vi "16T_Split_Cluster.vi"(0 "16 T Magnet control":T3={"Clamp"=FALSE, "Switch Heater"=FALSE, "Go to Zero"=FALSE, "Go to set"=FALSE, "Go to Hold"=FALSE, "Clamped"=FALSE, "Quenched"=FALSE, "Rate limit"=FALSE, "Persistent"=FALSE, "Hold"=FALSE, "Set"=FALSE, "Zero"=FALSE, "Magnet (T)"=0.0, "Leads (T)"=0.0, "Magnet T (K)"=3.4572, "Switch"=FALSE, "Setpoint (T)"=3.4572, "Rate (T/min)"=0.0, "Select"=FALSE, "Sweeping"=FALSE} {"Rate (T/min)" format="%6_5f"; "Setpoint (T)" format="%6_5f"; "Magnet T (K)" format="%6_5f"}) -> (1 "16 T Magnet control":T2={"Clamp"=FALSE, "Switch Heater"=FALSE, "Go to Zero"=FALSE, "Go to Set"=FALSE, "Go to Hold"=FALSE, "Setpoint (T)"=3.4572, "Rate (T/min)"=0.0, "Set Rate"=FALSE} {"Rate (T/min)" format="%6_5f"; "Setpoint (T)" format="%#4_5f"}, 2 "16 T Status":T1={"Clamped"=FALSE, "Quenched"=FALSE, "Rate limit"=FALSE, "Persistent"=FALSE, "Hold"=FALSE, "Set"=FALSE, "Zero"=FALSE, "Magnet (T)"=0.0, "Leads (T)"=0.0, "Magnet T (K)"=3.4572, "Switch"=FALSE, "Sweeping"=FALSE} {"Magnet T (K)" format="%#4_5f"; "Leads (T)" format="%6_5f"})   [LabVIEW 2019]
uses:
  S16/16T-Cluster.ctl
  S16/16T_Control.ctl
  S16/16T_Status.ctl
panel:
  # "20 T"
  # "20 T"
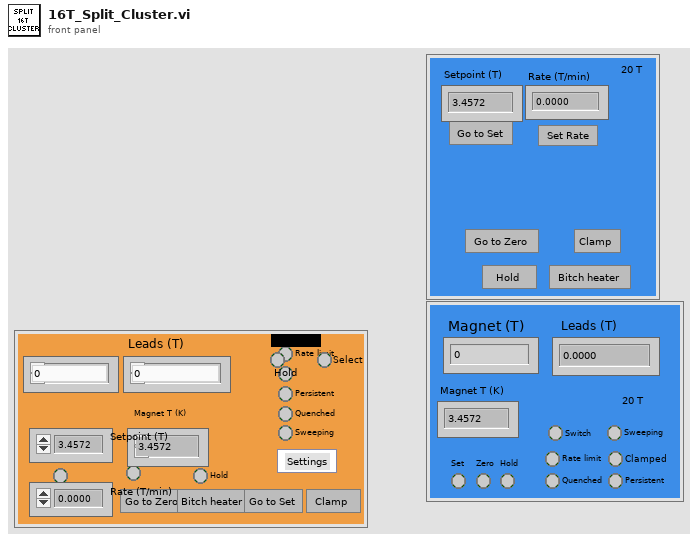
[diagram p1: front panel]
types:
  T1 = typedef "16T_Status.ctl" = cluster{"Clamped":bool, "Quenched":bool, "Rate limit":bool, "Persistent":bool, "Hold":bool, "Set":bool, "Zero":bool, "Magnet (T)":dbl, "Leads (T)":dbl, "Magnet T (K)":dbl, "Switch":bool, "Sweeping":bool}
  T2 = typedef "16T_Control.ctl" = cluster{"Clamp":bool, "Switch Heater":bool, "Go to Zero":bool, "Go to Set":bool, "Go to Hold":bool, "Setpoint (T)":dbl, "Rate (T/min)":dbl, "Set Rate":bool}
  T3 = typedef "16T-Cluster.ctl" = cluster{"Clamp":bool, "Switch Heater":bool, "Go to Zero":bool, "Go to set":bool, "Go to Hold":bool, "Clamped":bool, "Quenched":bool, "Rate limit":bool, "Persistent":bool, "Hold":bool, "Set":bool, "Zero":bool, "Magnet (T)":dbl, "Leads (T)":dbl, "Magnet T (K)":dbl, "Switch":bool, "Setpoint (T)":dbl, "Rate (T/min)":dbl, "Select":bool, "Sweeping":bool}
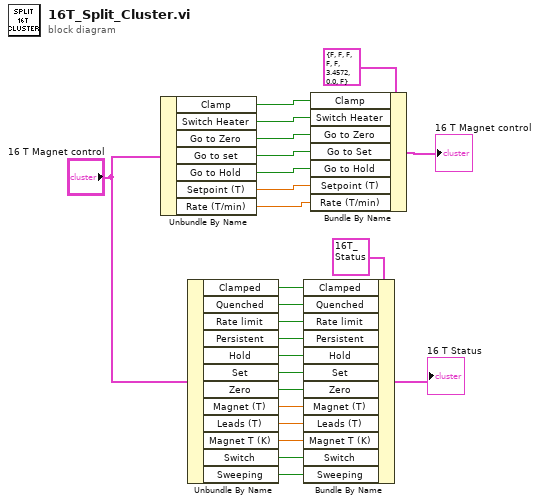
[diagram p0: block diagram]
diagram:
  n1 = Unbundle By Name("16 T Magnet control") -> ("Clamp"=w13:bool, "Switch Heater"=w12:bool, "Go to Zero"=w11:bool, "Go to set"=w10:bool, "Go to Hold"=w9:bool, "Setpoint (T)"=w8:dbl, "Rate (T/min)"=w7:dbl)
  n2 = Unbundle By Name("16 T Magnet control") -> ("Clamped"=w24:bool, "Quenched"=w23:bool, "Rate limit"=w22:bool, "Persistent"=w21:bool, "Hold"=w20:bool, "Set"=w19:bool, "Zero"=w18:bool, "Magnet (T)"=w17:dbl, "Leads (T)"=w16:dbl, "Magnet T (K)"=w15:dbl, "Switch"=w14:bool, "Sweeping"=w1:bool)
  n3 = Bundle By Name(cluster=T1 {"Clamped"=FALSE, "Quenched"=FALSE, "Rate limit"=FALSE, "Persistent"=FALSE, "Hold"=FALSE, "Set"=FALSE, "Zero"=FALSE, "Magnet (T)"=0.0, "Leads (T)"=0.0, "Magnet T (K)"=3.4572, "Switch"=FALSE, "Sweeping"=FALSE} ("20 T Magnet control 3"), "Clamped"=w24, "Quenched"=w23, "Rate limit"=w22, "Persistent"=w21, "Hold"=w20, "Set"=w19, "Zero"=w18, "Magnet (T)"=w17, "Leads (T)"=w16, "Magnet T (K)"=w15, "Switch"=w14, "Sweeping"=w1) -> (→"16 T Status":T1)
  n4 = Bundle By Name(cluster=T2 {"Clamp"=FALSE, "Switch Heater"=FALSE, "Go to Zero"=FALSE, "Go to Set"=FALSE, "Go to Hold"=FALSE, "Setpoint (T)"=3.4572, "Rate (T/min)"=0.0, "Set Rate"=FALSE} ("20 T Magnet control 2"), "Clamp"=w13, "Switch Heater"=w12, "Go to Zero"=w11, "Go to Set"=w10, "Go to Hold"=w9, "Setpoint (T)"=w8, "Rate (T/min)"=w7) -> (→"16 T Magnet control":T2)
